vi "Get Used J1939 Addresses.vi"(8 "error in (no error)":errorcluster, 11 "Node Ptr":u64) -> (0 "error out":errorcluster, 2 "Addresses":u8[](array[numeric]), 3 "Item Ref out":T1 format="%.0x")   [LabVIEW 2013, in "J1939 Addon System Explorer.lvlib"]
uses:
  J1939 Addon System Explorer.lvlib
  <vilib>/NI Veristand/Custom Device API/Custom Device Item Ref.ctl
  <vilib>/NI Veristand/Custom Device Tools/Custom Device Utility Library/Search Direction.ctl
  Shared/Types/Monitor Settings.ctl
  Shared/SubVIs/Constants.vi
  <vilib>/NI Veristand/Custom Device Tools/Custom Device Utility Library/NI VeriStand - Search for Item by GUID.vi
  <vilib>/NI Veristand/Custom Device Tools/Custom Device Utility Library/NI VeriStand - Search for All Items by GUID.vi
  <vilib>/NI Veristand/Custom Device API/Get Item Property (Variant).vi
  Shared/J1939 Addon Shared.lvlib
  <vilib>/NI Veristand/Custom Device API/Custom Device API.lvlib
  <vilib>/NI Veristand/Custom Device Tools/Custom Device Utility Library/Custom Device Utility Library.lvlib
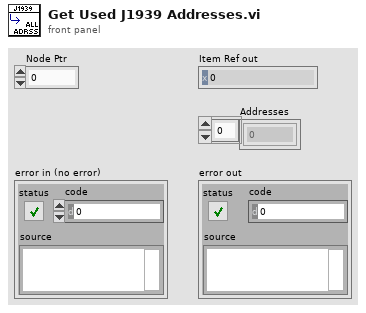
[diagram p1: front panel]
types:
  T1 = typedef "Custom Device API.lvlib/Custom Device Item Ref.ctl" = u64
  T2 = typedef "Custom Device Utility Library.lvlib/Search Direction.ctl" = enum16{"Down", "Up"}
  T3 = typedef "J1939 Addon Shared.lvlib/Monitor Settings.ctl" = cluster{"J1939 Network Address":u8, "Name":u64}
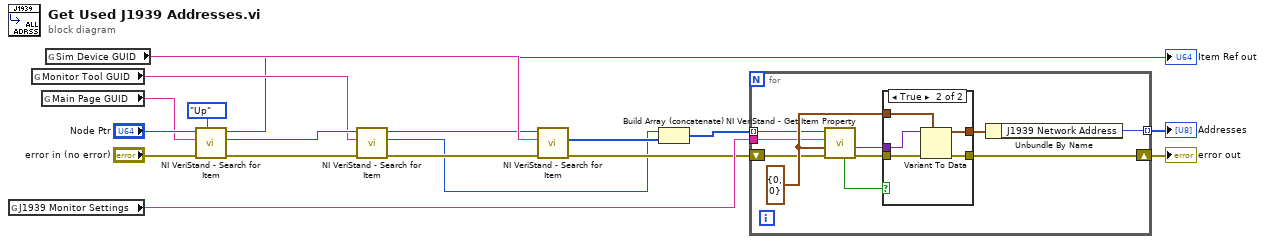
[diagram p0: block diagram]
diagram:
  n1 = global read "Constants.vi" "J1939 Monitor Settings"() -> (w17:string)
  n2 = global read "Constants.vi" "Monitor Tool GUID"() -> (w6:string)
  n3 = global read "Constants.vi" "Main Page GUID"() -> (w10:string)
  n4 = global read "Constants.vi" "Sim Device GUID"() -> (w14:string)
  n5 = call-poly <vilib>:"NI VeriStand - Search for Item.vi"("Direction (Down)"=Search_Direction."Up", "error in"="error in (no error)", "Item GUID"=w10, "Section Ref in"="Node Ptr") -> ("error out"=w8:errorcluster, "Item Ref"=w9:T1, "Section Ref out"=→"Item Ref out":T1)  [unwired: 4 in, 1 out]
  n6 = call-poly <vilib>:"NI VeriStand - Search for Item.vi"("error in"=w8, "Item GUID"=w6, "Section Ref in"=w9) -> ("error out"=w7:errorcluster, "Item Ref"=w4:T1, "Section Ref out"=w2:T1)  [unwired: 5 in, 1 out]
  n7 = call-poly <vilib>:"NI VeriStand - Search for Item.vi"("error in"=w7, "Item GUID"=w14, "Section Ref in"=w2) -> ("error out"=w15:errorcluster, "Item Refs"=w5:T1[])  [unwired: 5 in, 2 out]
  n8 = Build Array (concatenate)(w4, w5) -> (w3:T1[])
  n9 = for {
    shift-right: [w22] -> w16
    shift-left: w15 -> [w23]
    tunnel: w17 -> [w21]
    tunnel: w3 -> [w20] mode=indexing
    tunnel: [w19] -> w18 mode=indexing
    w27 = T3 {"J1939 Network Address"=0, "Name"=0} ("J1939 XNET Settings")
    n10 = call-poly <vilib>:"NI VeriStand - Get Item Property.vi"("error in (no error)"=w23, "Default Value"=w27, "Property Name"=w21, "Item Ref in"=w20) -> ("error out"=w24:errorcluster, "Value"=w25:variant, "Found?"=w26:bool)  [unwired: 4 in, 1 out]
    n11 = case shown="True" w26 {
      tunnel: w24 -> [w30 w35]
      tunnel: [w30 w34] -> w22
      tunnel: w25 -> [_ w33]
      tunnel: w27 -> [w29 w32]
      tunnel: [w29 w31] -> w28
      frame False {
      }
      frame True {
        n12 = Variant To Data(error in=w35, type=w32, Variant=w33) -> (data=w31:T3, error out=w34:errorcluster)
      }
    }
    n13 = Unbundle By Name(w28) -> ("J1939 Network Address"=w19:u8)
  }
  "Addresses" <- w18
  "error out" <- w16
